vi "Example.vi"() -> ()   [LabVIEW 2020]
doc: "Example of simple uses class in LabVIEW. Comments in Polish."
uses:
  Jedi/Jedi.lvclass
  Droid/Droid.lvclass
panel:
  in  "Slide":dbl(slide) scale=0.0..10.0
  out "Error Out":errorcluster
  in  "Jedi.lvclass":refnum<class "Jedi.lvclass">
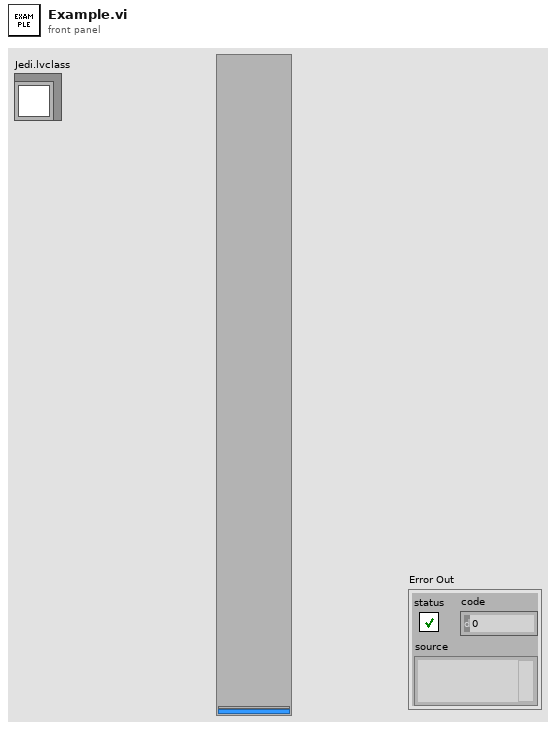
[diagram p1: front panel]
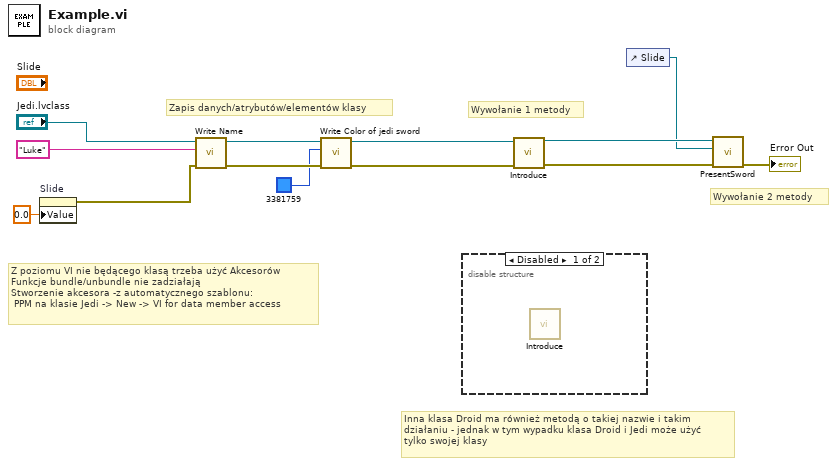
[diagram p0: block diagram]
diagram:
  # "Inna klasa Droid ma również metodą o takiej nazwie i takim \ndziałaniu - jednak w tym wypadku klasa Droid i Jedi może użyć\ntylko swojej klasy"
  # "Wywołanie 2 metody"
  # "Wywołanie 1 metody"
  # "Z poziomu VI nie będącego klasą trzeba użyć Akcesorów\nFunkcje bundle/unbundle nie zadziałają\nStworzenie akcesora -z automatycznego szablonu:\n PPM na klasie Jedi -> New -> VI for data member access"
  # "Zapis danych/atrybutów/elementów klasy"
  n1 = property on="Slide" class="Slide (strict)"("Value"=0.0 ("Slide")) -> (error out=w2:errorcluster)  [unwired: 2 in, 1 out]
  n2 = call-dynamic "Write Name.vi"("error in (no error)"=w2, "Name"="Luke", "Jedi in"="Jedi.lvclass") -> ("error out"=w8:errorcluster, "Jedi out"=w6:refnum<class "Jedi.lvclass">)  [unwired: 7 in]
  n3 = call-dynamic "Write Color of jedi sword.vi"("error in (no error)"=w8, "Color of jedi sword"=u32 3381759, "Jedi in"=w6) -> ("error out"=w7:errorcluster, "Jedi out"=w5:refnum<class "Jedi.lvclass">)  [unwired: 7 in]
  n4 = disable-structure shown="Disabled" {
    frame Disabled {
      n5 = call-dynamic "Introduce.vi"() -> ()  [unwired: 10 in, 2 out]
    }
    frame Enabled {
    }
  }
  n6 = call-dynamic "Introduce.vi"("Error In"=w7, "Jedi in"=w5) -> ("Error Out"=w11:errorcluster, "Jedi out"=w10:refnum<class "Jedi.lvclass">)  [unwired: 8 in]
  n7 = control-ref of="Slide"() -> (w4:refnum<vi>)
  n8 = call-dynamic "PresentSword.vi"("Error In"=w11, "Slide Refnum"=w4, "Jedi in"=w10) -> ("Error Out"=→"Error Out":errorcluster)  [unwired: 7 in, 1 out]
